vi "Read Admin Enable.vi"(8 "error in (no error)":errorcluster, 11 "Master in":refnum<class "Master.lvclass">) -> (0 "error out":errorcluster, 1 "User Enable":bool, 2 "Admin Enable":bool, 3 "Master out":refnum<class "Master.lvclass">, 4 "Cancle 3":bool, 5 "User Name 2":string)   [LabVIEW 2014, in "Master.lvclass"]
uses:
  Master/Master.lvclass
  Master/Master.lvclass/Master.ctl
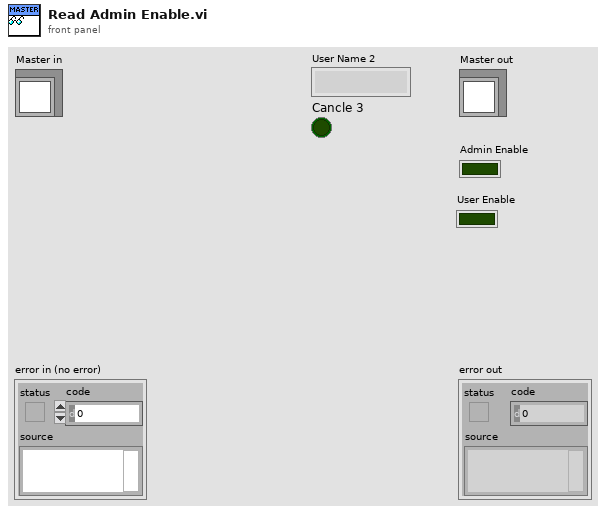
[diagram p1: front panel]
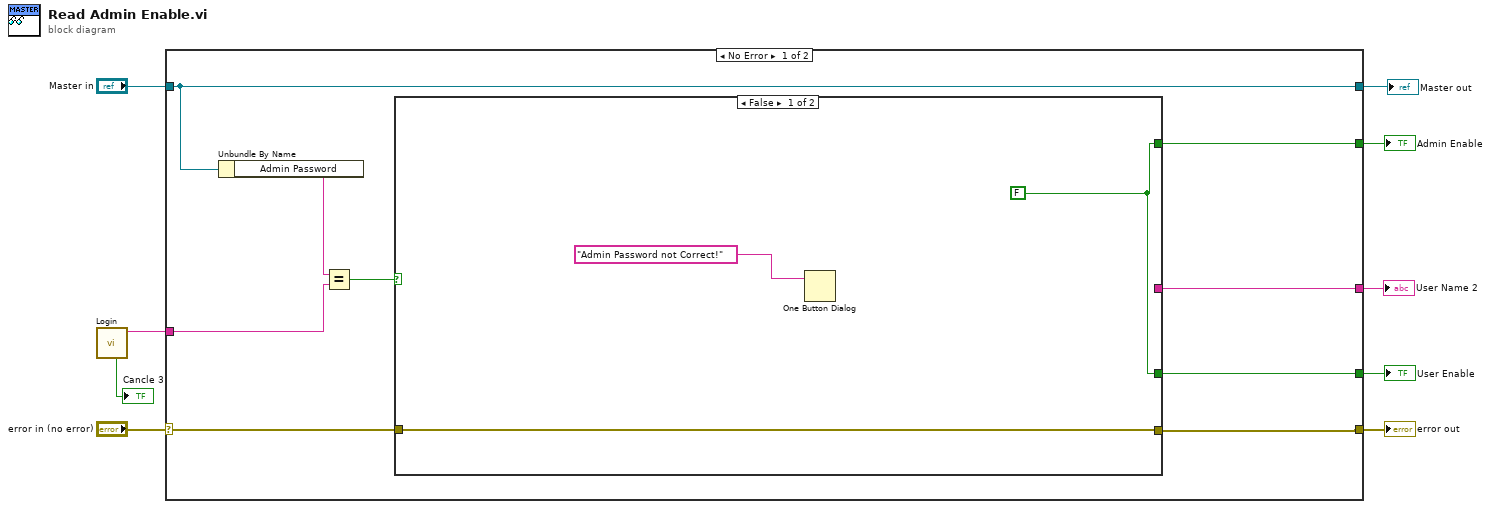
[diagram p0: block diagram]
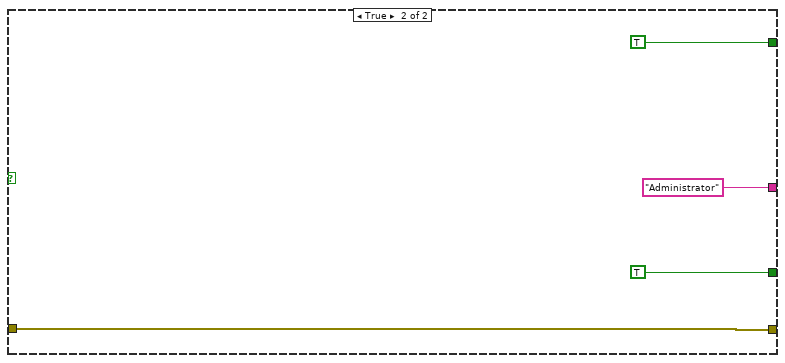
[diagram p2: hidden frame]
diagram:
  n1 = call "Login.vi"() -> ("Login Password 2"=w3:string, "Cancle"=→"Cancle 3":bool)  [unwired: 9 in, 1 out]
  n2 = case shown="No Error" "error in (no error)" {
    selector: "error in (no error)" -> [w14 w27]
    tunnel: [w13 w27] -> w5
    tunnel: [w15 w26] -> w7
    tunnel: "Master in" -> [w15 w26]
    tunnel: w3 -> [w11 _]
    tunnel: [w18 _] -> w6
    tunnel: [w17 _] -> w4
    tunnel: [w16 _] -> w2
    frame No Error {
      n3 = Unbundle By Name(w15) -> ("Admin Password"=w10:string)
      n4 = Equal?(x=w10, y=w11) -> (x = y?=w12:bool)
      n5 = case shown="False" w12 {
        tunnel: [w20 TRUE ("Admin Enable")] -> w18
        tunnel: [w20 TRUE ("User Enable")] -> w17
        tunnel: [_ "Administrator" ("User Name 2")] -> w16
        tunnel: w14 -> [w21 w22]
        tunnel: [w21 w22] -> w13
        frame False {
          w20 = FALSE
          n6 = One Button Dialog(message="Admin Password not Correct!") -> ()  [unwired: 1 in, 1 out]
        }
        frame True {
        }
      }
    }
    frame Error {
    }
  }
  "error out" <- w5
  "Master out" <- w7
  "Admin Enable" <- w6
  "User Enable" <- w4
  "User Name 2" <- w2
